vi "Measurement UI.vi"() -> ()   [LabVIEW 2023, in "FPT_Compression UI.lvlib"]
uses:
  FPT_Compression UI.lvlib
panel:
  in  "Measurement Graph":T1(tab)
  out "General Graph 1":T2(graph)
  out "General Graph 2":T2(graph)
  out "General Graph 3":T2(graph)
  out "General Graph 4":T2(graph)
  out "General Graph 5":T2(graph)
  out "PAE@Pin(s)":string[](array[string])
  out "Gain@Pin(s)":string[](array[string])
  out "Pout@Pin(s)":string[](array[string])
  out "Pout@Pin vs Freq":dbl[][](array[numeric])
  out "PAE vs Pin per Freq":dbl[][](array[numeric])
  in  "RFSG attenuation s2p path name":string caption="RFSG ATTENUATION S2P PATH NAME"
  in  "RFmx attenuation s2p path name":string caption="RFmx ATTENUATION S2P PATH NAME"
  in  "RFSG attenuation path name":string caption="RFSG ATTENUATION PATH NAME"
  in  "RFmx attenuation path name":string caption="RFmx ATTENUATION PATH NAME"
  out "Gain vs Pin per Freq":dbl[][](array[numeric])
  out "Group B Graph":refnum<vi>[](array[refnum])
  out "Group A Graph":refnum<vi>[](array[refnum])
  in  "Power sequencing file path":string
  in  "RFSG name":string="5842_0"
  in  "RFSG attenuation mode":T3(ring)=enum."s2p File"
  in  "RFSG s2p file path":string
  in  "RFmx name":string="5842_0"
  in  "RFmx attenuation mode":T3(ring)=enum."Constant Attenuation"
  in  "RFmx s2p file path":string
  out "All Graph Refs":refnum<vi>[](array[refnum])
  out "Pout vs Pin per Freq":dbl[][](array[numeric])
  out "OPxdB vs Freq":dbl[][](array[numeric])
  out "Linear Gain vs Freq":dbl[][](array[numeric])
  out "Frequencies":string[](array[string])
  out "OPxdB(s)":string[](array[string])
  out "Linear Gain(s)":string[](array[string])
  out "Full Data per Frequency":string[][](array[string])
  out "Pin(s)":string[](array[string])
  in  "Compression_Stimulus Mode":T4(ring)
  in  "SMU name":string caption="SMU Name"
  out "Table 2 Header":string[](array[string])
  out "Table 1 Header":string[](array[string])
  out "Gain@Pin vs Freq":dbl[][](array[numeric])
  out "PAE@Pin vs Freq":dbl[][](array[numeric])
  out "MeasTable 1":string[][](table)
  out "MeasTable 2":string[][](table)
  in  "Mode of operation":T5(ring) caption="Configuration"
  in  "Tab Control":T6(tab)
  in  "Power sequencing file path_update":path caption="Power Sequencing File Path"
  in  "SMU channel":string caption="SMU Channel"
  in  "SMU name_update":refnum<k15> caption="SMU Name"
  in  "RFmx port":string(combo)="port2" caption="RFmx Port"
  in  "RFSG port":string(combo)="port1" caption="RFSG Port"
  in  "RFSG name_update":refnum<k15> caption="RFSG Name"
  in  "RFSG attenuation mode_tab":T3(tab)=enum."s2p File" caption="RFSG Attenuation Mode"
  in  "RFSG external attenuation (dB)":dbl caption="External Attenuation" format="%#.3fdB"
  in  "RFSG s-parameters orientation":enum32{"Port1 Towards DUT", "Port2 Towards DUT"}(ring) caption="Orientation"
  in  "RFSG s2p file path_update":path caption="S2P File Path"
  in  "RFmx attenuation mode_tab":T3(tab)=enum."s2p File" caption="RFmx Attenuation Mode"
  in  "RFmx external attenuation (dB)":dbl caption="External Attenuation" format="%#.3fdB"
  in  "RFmx s2p file path_update":path caption="S2P File Path"
  in  "RFmx s-parameters orientation":enum32{"Port1 Towards DUT", "Port2 Towards DUT"}(ring) caption="Orientation"
  in  "RFmx name_update":refnum<k15> caption="RFmx Name"
  in  "DC & RF Mode":T4(tab)
  in  "CP_CW_DC Source Delay (s)":dbl caption="DC Source Delay" format="%#ps"
  in  "CP_PRF_RFmx Trigger Delay (s)":dbl caption="RFmx Trigger Delay" format="%#ps"
  in  "CP_PRF_PRI (s)":dbl=0.001 caption="PRI" format="%#ps"
  in  "CP_PRF_RF Pulse Width (s)":dbl=0.0001 caption="RF Pulse Width" format="%#ps"
  in  "CP_PRF_DC Source Delay (s)":dbl caption="DC Source Delay" format="%#ps"
  in  "PP_PRF_ON Current Limit (A)":dbl=0.2 caption="Pulse ON Current Limit" format="%#pA"
  in  "PP_PRF_PRI (s)":dbl=0.001 caption="PRI" format="%#ps"
  in  "PP_PRF_RF Pulse Width (s)":dbl=0.0001 caption="RF Pulse Width" format="%#ps"
  in  "PP_PRF_DC Source Delay (s)":dbl caption="DC Source Delay" format="%#ps"
  in  "PP_PRF_RFmx Trigger Delay (s)":dbl caption="RFmx Trigger Delay" format="%#ps"
  in  "PP_PRF_DC Pulse Width (s)":dbl=0.0008 caption="DC Pulse Width" format="%#ps"
  in  "PP_PRF_Bias Voltage Level (V)":dbl caption="Pulse OFF Voltage Level" format="%#pV"
  in  "PP_PRF_Bias Current Limit (A)":dbl=0.2 caption="Pulse OFF Current Limit" format="%#pA"
  in  "Compression_DC Measurement Interval (s)":dbl=5e-05 caption="DC Measurement Interval" format="%#ps"
  in  "Compression_RF Measurement Interval (s)":dbl=5e-05 caption="RF Measurement Interval" format="%#ps"
  in  "Compression_Target Pin (dBm)":dbl=1.0 caption="Target Pin" format="%#pdBm"
  in  "Compression_Expected DUT Gain (dB)":dbl=17.5 caption="Expected DUT Gain" format="%#pdB"
  in  "Compression_Max Linear Range (dBm)":dbl=-10.0 caption="Max Linear Range" format="%#pdBm"
  in  "Compression_Compression Point (dB)":dbl=1.0 caption="PxdB" format="%#pdB"
  in  "Compression_RFSG Frequency Start (Hz)":dbl=6000000000.0 caption="Frequency Start" step=1000000.0 format="%#pHz"
  in  "Compression_RFSG Power Start (dBm)":dbl=-20.0 caption="Power Start" format="%#pdBm"
  in  "Compression_RFSG Power Step Size (dB)":dbl=1.0 caption="Power Step Size" format="%#pdB"
  in  "Compression_RFSG Power Stop(dBm)":dbl=4.0 caption="Power End" format="%#pdBm"
  in  "Compression_RBW (Hz)":dbl=5000000.0 caption="RBW" format="%#pHz"
  in  "Compression_RFSG Frequency Stop (Hz)":dbl=18000000000.0 caption="Frequency Stop" step=1000000.0 format="%#pHz"
  in  "Compression_RFSG Number of Frequency Step":i32=10 caption="Number of Steps"
  out "Status":string
  # "Frequency Sweep"
  # "Power Sweep"
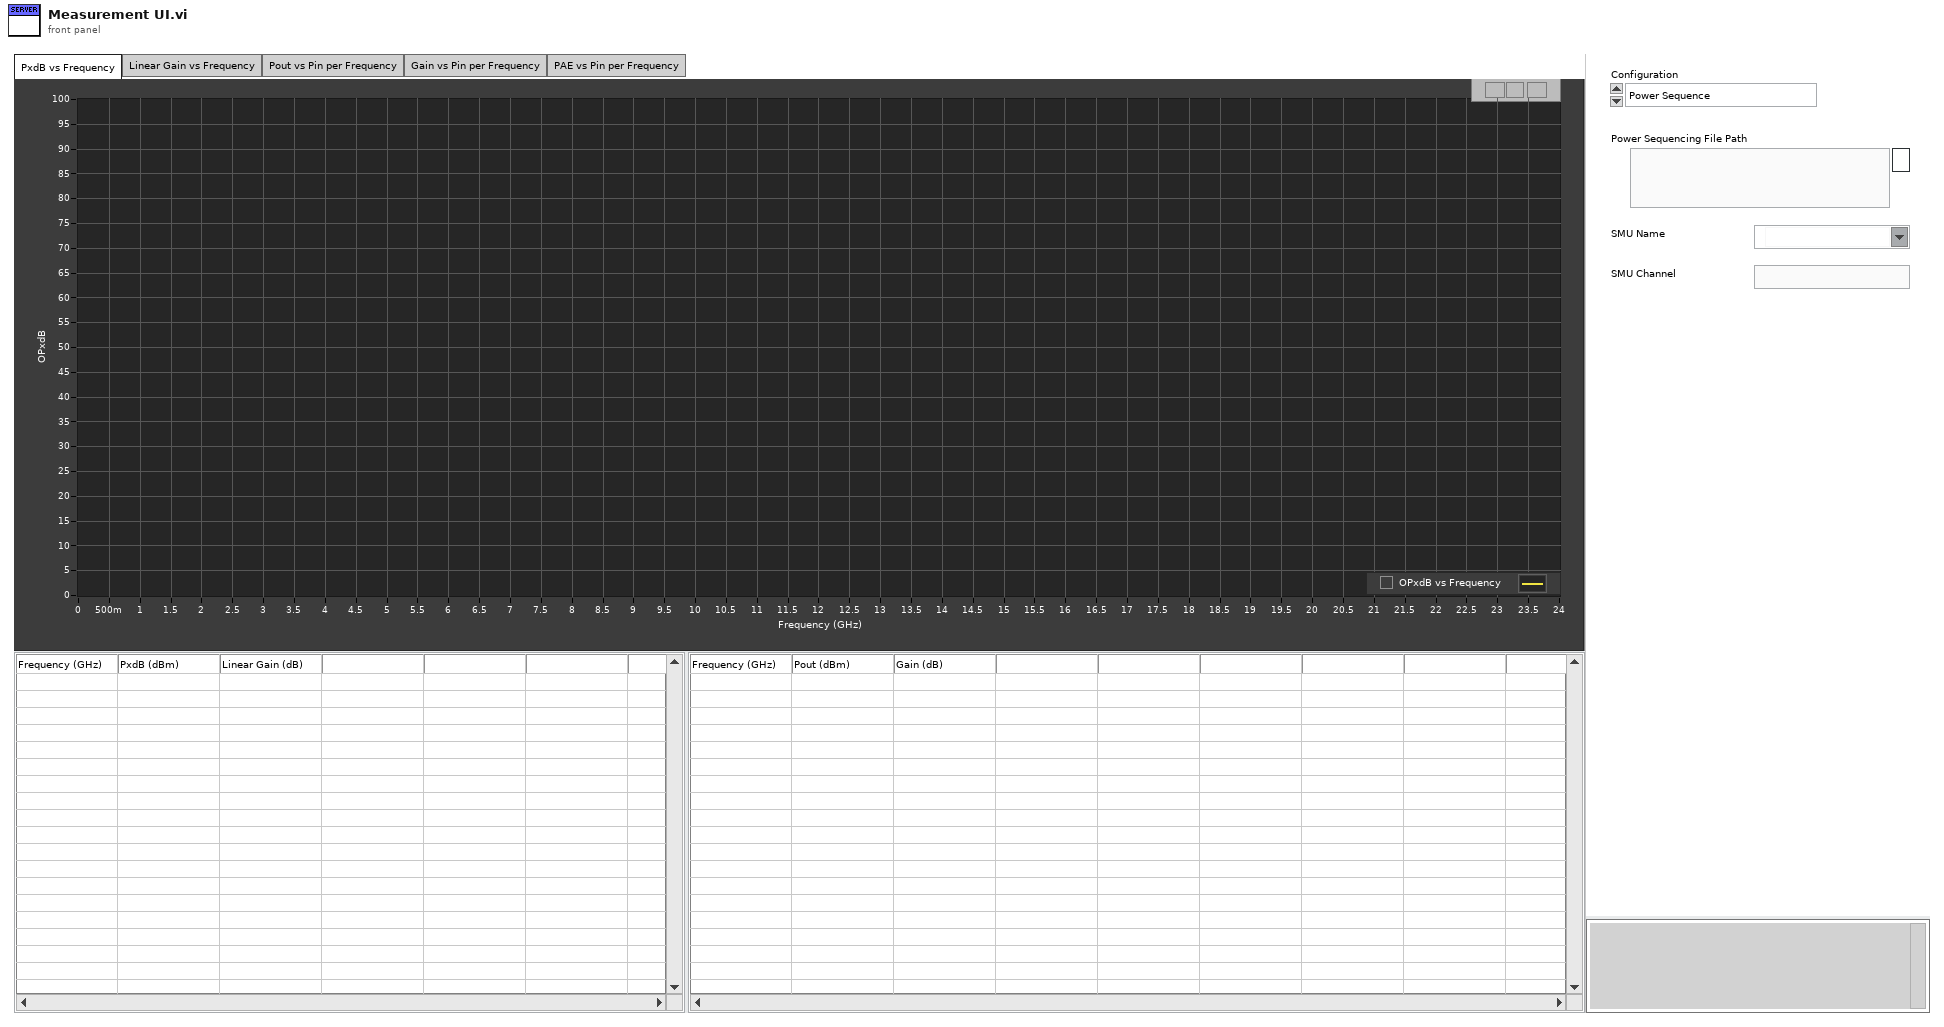
[diagram p1: front panel]
types:
  T1 = enum32{"PxdB vs Frequency", "Linear Gain vs Frequency", "Pout vs Pin per Frequency", "Gain vs Pin per Frequency", "PAE vs Pin per Frequency", "Hidden Controls"}
  T2 = cluster{"Load currents":dbl[], "Efficiency":dbl[]}[]
  T3 = enum32{"<None>", "Constant Attenuation", "s2p File"}
  T4 = enum32{"Constant Power and RF", "Constant Power and Pulsed RF", "Pulsed Power and RF"}
  T5 = enum32{"Power Sequence", "HW + Correction", "Mode", "Measurement 1"}
  T6 = enum32{"Power Sequence", "Correction", "Mode", "Measurement 1"}
  T7 = enum16{"<None>", "Constant Attenuation", "s2p File"}
  T8 = cluster{"Shift":bool, "Ctrl":bool, "Alt":bool, "Cmd":bool, "Opt":bool}
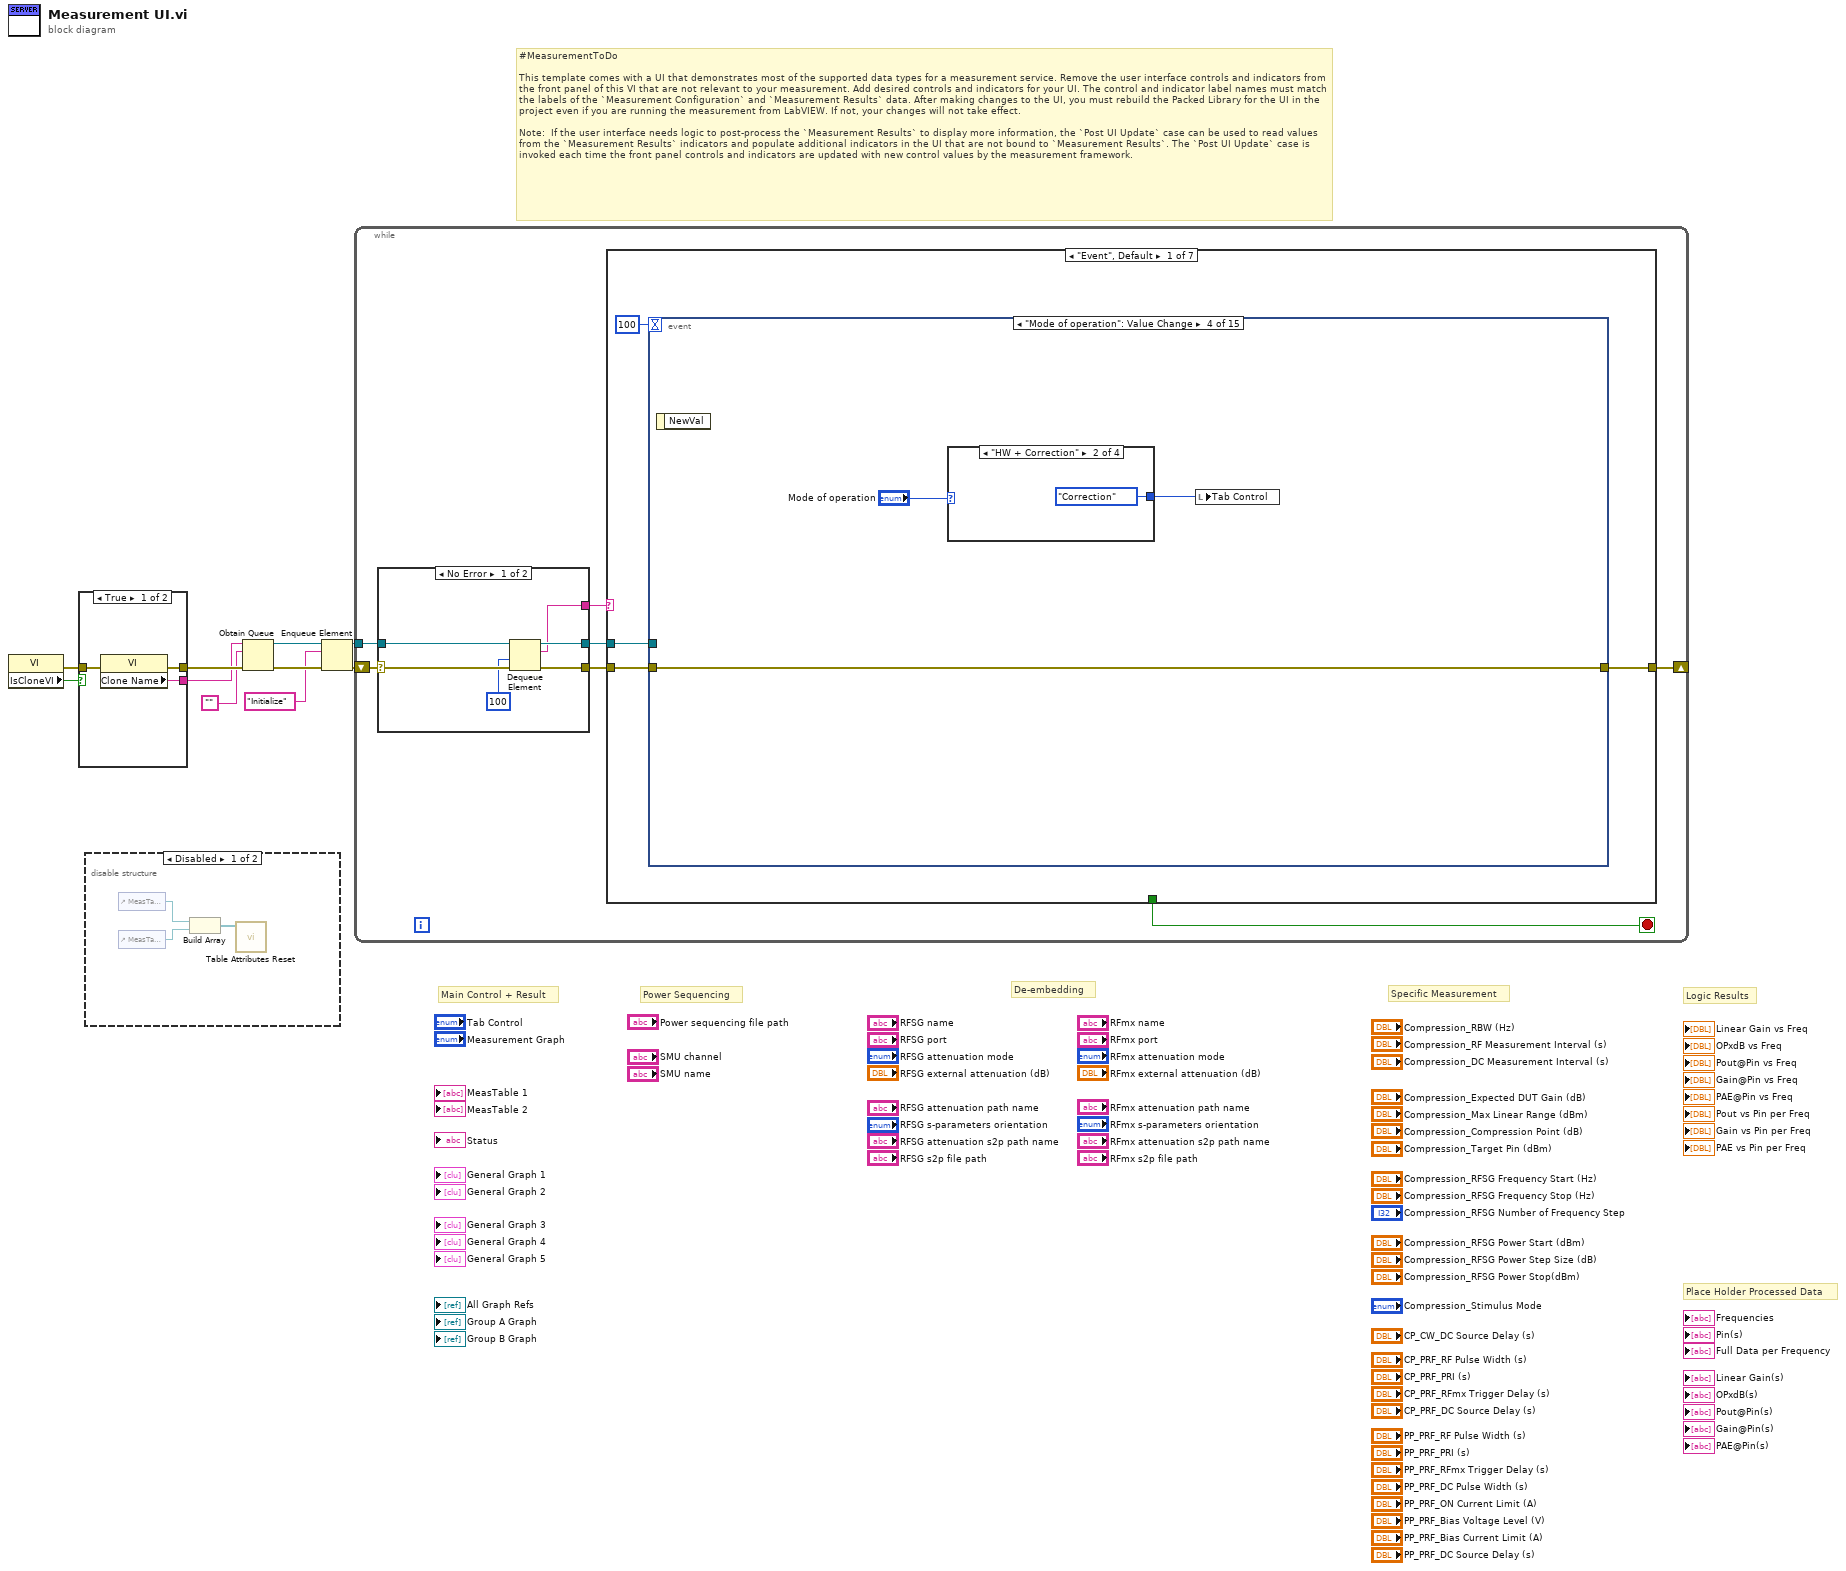
[diagram p0: block diagram]
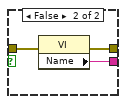
[diagram p3: hidden frame]
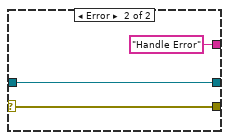
[diagram p4: hidden frame]
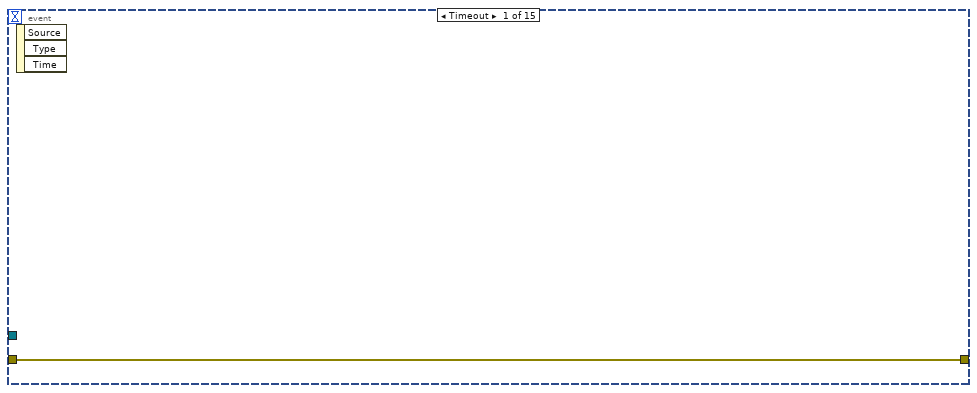
[diagram p5: hidden frame]
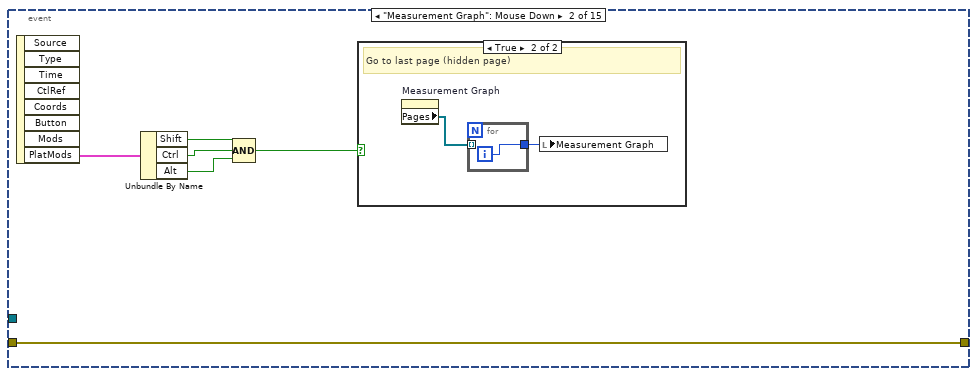
[diagram p6: hidden frame]
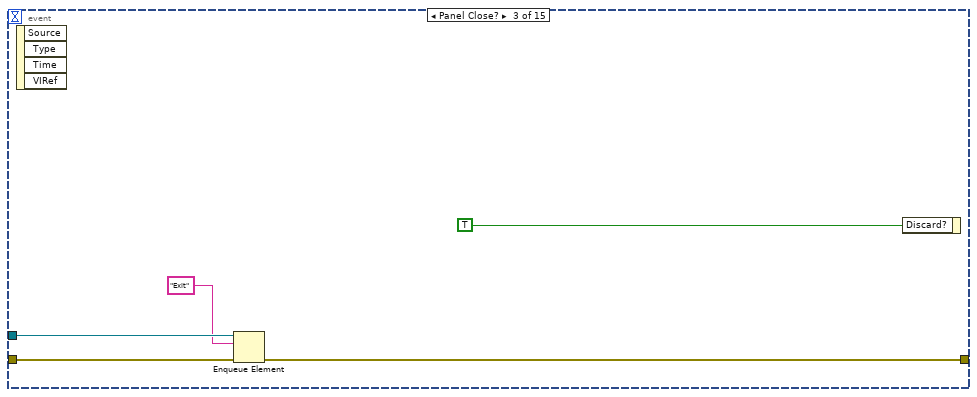
[diagram p8: hidden frame]
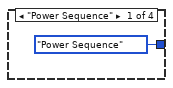
[diagram p9: hidden frame]
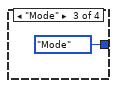
[diagram p10: hidden frame]
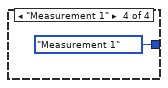
[diagram p11: hidden frame]
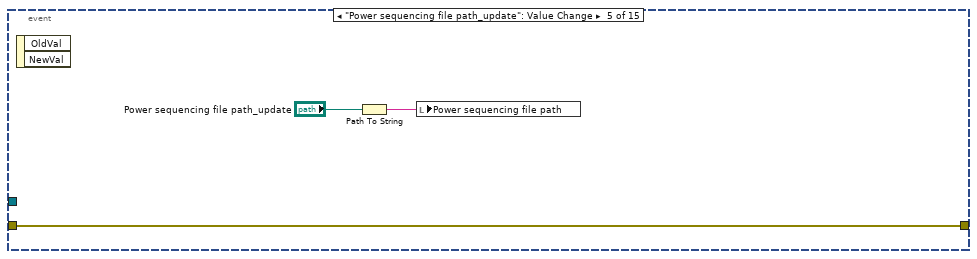
[diagram p12: hidden frame]
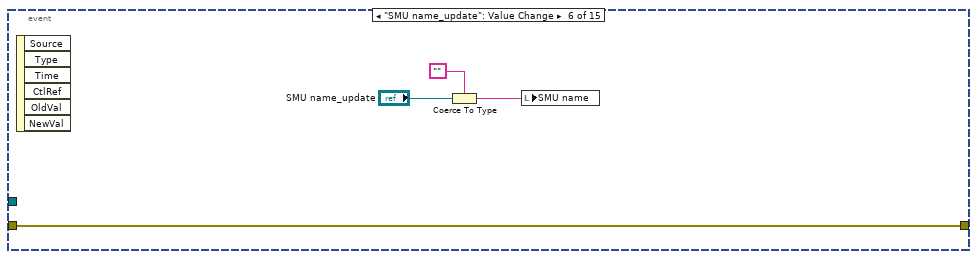
[diagram p13: hidden frame]
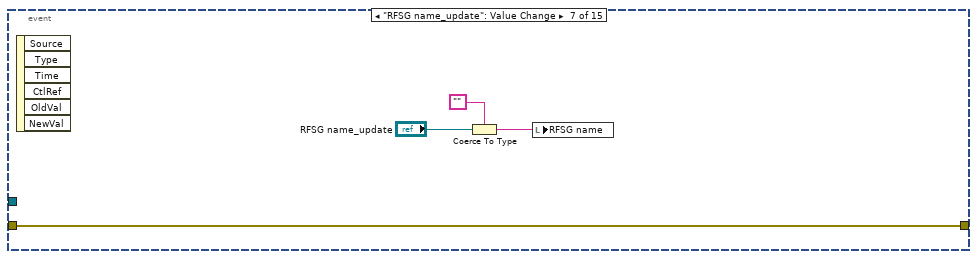
[diagram p14: hidden frame]
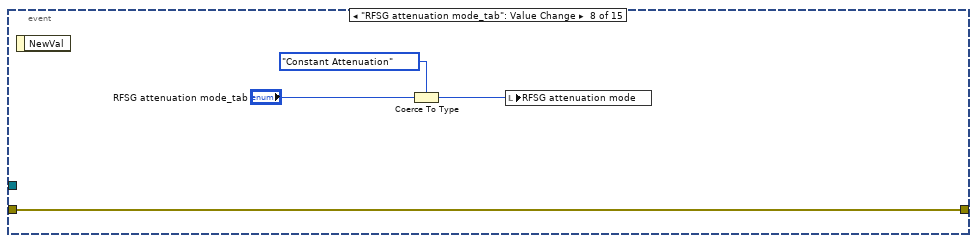
[diagram p15: hidden frame]
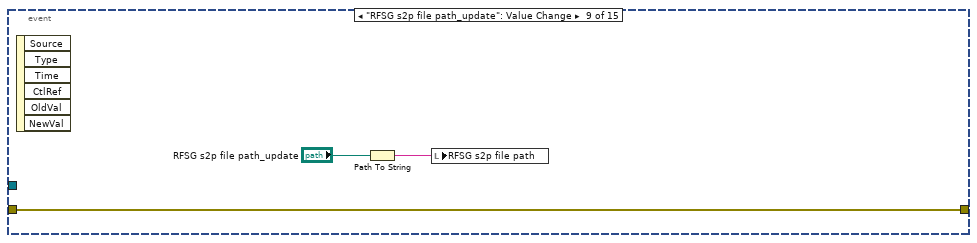
[diagram p16: hidden frame]
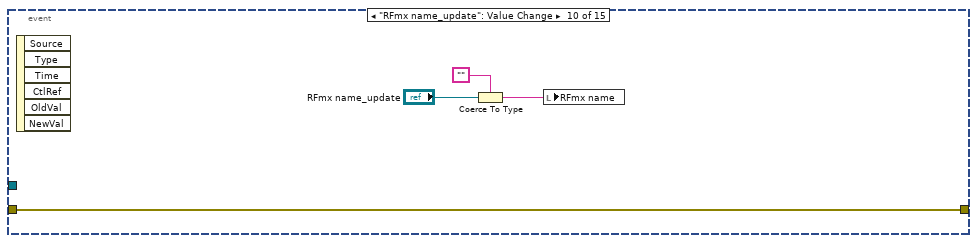
[diagram p17: hidden frame]
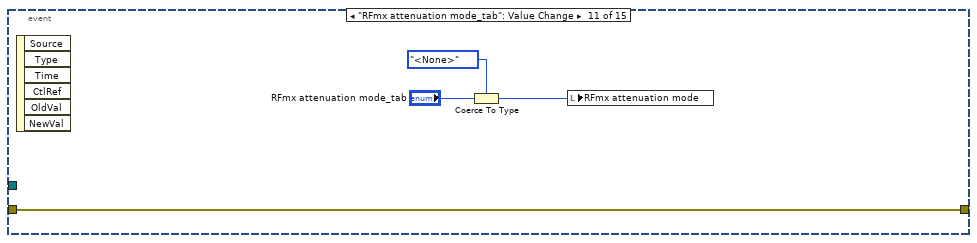
[diagram p18: hidden frame]
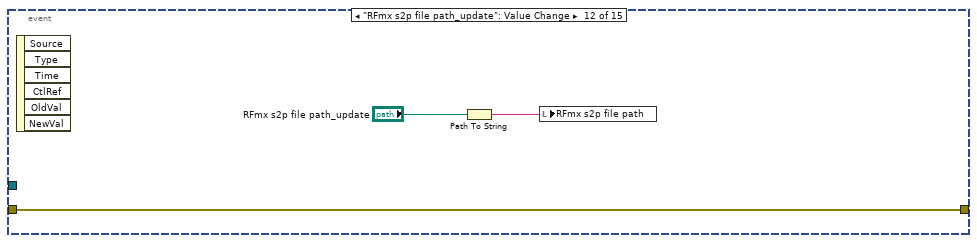
[diagram p19: hidden frame]
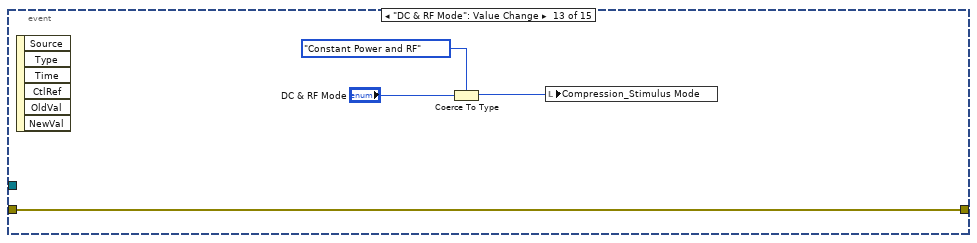
[diagram p20: hidden frame]
diagram:
  # "Logic Results"
  # "Place Holder Processed Data"
  # "Specific Measurement"
  # "De-embedding"
  # "Power Sequencing"
  # "Main Control + Result"
  # "#MeasurementToDo  \n\nThis template comes with a UI that demonstrates most of the supported data types for a measurement service. Remove the user interface controls and indicators from the front panel of this VI that are not relevant to your measurement. Add desired controls and indicators for your UI. The control and indicator label names must match the labels of the `Measurement Configuration` and `Measurement Results` data. After making changes to the UI, you must rebuild the Packed Library for the UI in the project even if you are running the measurement from LabVIEW. If not, your changes will not take effect.\n\nNote:  If the user interface needs logic to post-process the `Measurement Results` to display more information, the `Post UI Update` case can be used to read values from the `Measurement Results` indicators and populate additional indicators in the UI that are not bound to `Measurement Results`. The `Post UI Update` case is invoked each time the front panel controls and indicators are updated with new control values by the measurement framework."
  n1 = property class="VI"() -> (error out=w1:errorcluster, "IsCloneVI"=w2:bool)  [unwired: 2 in, 1 out]
  n2 = case shown="True" w2 {
    tunnel: [w13 w16] -> w10
    tunnel: [w12 w15] -> w9
    tunnel: w1 -> [w11 w14]
    frame True {
      n3 = property class="VI"(error in=w11) -> (error out=w13:errorcluster, "Clone Name"=w12:string)  [unwired: 1 in, 1 out]
    }
    frame False {
      n4 = property class="VI"(error in=w14) -> (error out=w16:errorcluster, "Name"=w15:string)  [unwired: 1 in, 1 out]
    }
  }
  n5 = disable-structure shown="Disabled" {
    frame Disabled {
      n6 = control-ref of="MeasTable 2"() -> (w19:refnum<vi>)
      n7 = control-ref of="MeasTable 1"() -> (w18:refnum<vi>)
      n8 = Build Array(w19, w18) -> (w17:refnum<vi>[])
      n9 = call "Table Attributes Reset.vi"("Table Refs"=w17) -> ()  [unwired: 11 in]
    }
    frame Enabled {
    }
  }
  n10 = Obtain Queue(name (unnamed)=w9, element data type="", error in (no error)=w10) -> (queue out=w6:refnum<queue>, error out=w8:errorcluster)  [unwired: 2 in, 1 out]
  n11 = Enqueue Element(queue=w6, element="Initialize", error in (no error)=w8) -> (queue out=w5:refnum<queue>, error out=w7:errorcluster)  [unwired: 1 in, 1 out]
  n12 = while {
    shift-right: [w21] -> _
    shift-left: w7 -> [w26]
    tunnel: w5 -> [w24]
    stop <- w20 stop-if-true
    n13 = case shown="No Error" w26 {
      selector: w26 -> [w32 w35]
      tunnel: [w31 w35] -> w25
      tunnel: w24 -> [w30 w34]
      tunnel: [w29 w34] -> w23
      tunnel: [w28 "Handle Error"] -> w22
      frame No Error {
        n14 = Dequeue Element(queue=w30, timeout in ms (-1)=100, error in (no error)=w32) -> (queue out=w29:refnum<queue>, element=w28:string, error out=w31:errorcluster)  [unwired: 1 out]
      }
      frame Error {
      }
    }
    n15 = case shown="\"Event\", Default" w22 {
      tunnel: w25 -> [w38 w150 w217 w259 w267 w274 w275]
      tunnel: w23 -> [w36 _ w216 w257 _ w272 _]
      tunnel: [w39 w150 w217 w258 w262 w269 w275] -> w21
      tunnel: [_ _ _ _ _ TRUE _] -> w20
      frame "Event", Default {
        n16 = event shown="[3] \"Mode of operation\": Value Change" {
          selector: _ -> [_ _ _ _ _ _ _ _ _ _ _ _ _ _ _]
          dyn-events: _ -> [_ _ _ _ _ _ _ _ _ _ _ _ _ _ _]
          timeout: 100 -> [_ _ _ _ _ _ _ _ _ _ _ _ _ _ _]
          tunnel: [w40 w41 w52 w56 w62 w68 w69 w73 w77 w80 w84 w88 w94 w107 w128] -> w39
          tunnel: w38 -> [w40 w41 w53 w56 w62 w68 w69 w73 w77 w80 w84 w88 w94 w109 w129]
          tunnel: w36 -> [_ _ w51 _ _ _ _ _ _ _ _ _ _ _ _]
          event Timeout {
            n17 = event-data() -> ()  [unwired: 1 in, 3 out]
          }
          event "Measurement Graph": Mouse Down {
            n18 = event-data() -> ("PlatMods"=w46:T8)  [unwired: 1 in, 7 out]
            n19 = Unbundle By Name(w46) -> ("Shift"=w45:bool, "Ctrl"=w44:bool, "Alt"=w43:bool)
            n20 = Compound Arithmetic op=AND(w45, w44, w43) -> (w42:bool)
            n21 = case shown="True" w42 {
              frame False {
              }
              frame True {
                # "Go to last page (hidden page)"
                n22 = property on="Measurement Graph" class="TabCtl (strict)"() -> ("Pages"=w48:refnum<vi>[])  [unwired: 2 in, 2 out]
                n23 = for {
                  tunnel: w48 -> [_] mode=indexing
                  tunnel: [w49] -> w47
                  i -> [w49]
                }
                n24 = local write "Measurement Graph"(w47) -> ()
              }
            }
          }
          event Panel Close? {
            n25 = event-data() -> ()  [unwired: 1 in, 4 out]
            n26 = Enqueue Element(queue=w51, element="Exit", error in (no error)=w53) -> (error out=w52:errorcluster)  [unwired: 1 in, 2 out]
            n27 = event-data("Discard?"=TRUE) -> ()  [unwired: 1 in, 1 out]
          }
          event "Mode of operation": Value Change {
            n28 = event-data() -> ()  [unwired: 1 in, 1 out]
            n29 = case shown="\"HW + Correction\"" "Mode of operation" {
              tunnel: [T6."Power Sequence" ("Tab Control") T6."Correction" ("Tab Control") T6."Mode" ("Tab Control") T6."Measurement 1" ("Tab Control")] -> w55
              frame "Power Sequence" {
              }
              frame "HW + Correction" {
              }
              frame "Mode" {
              }
              frame "Measurement 1" {
              }
            }
            n30 = local write "Tab Control"(w55) -> ()
          }
          event "Power sequencing file path_update": Value Change {
            n31 = event-data() -> ()  [unwired: 1 in, 2 out]
            n32 = Path To String(path="Power sequencing file path_update") -> (string=w63:string)
            n33 = local write "Power sequencing file path"(w63) -> ()
          }
          event "SMU name_update": Value Change {
            n34 = event-data() -> ()  [unwired: 1 in, 6 out]
            n35 = Coerce To Type(0:"SMU name_update", 1:"") -> (2:w65:string)
            n36 = local write "SMU name"(w65) -> ()
          }
          event "RFSG name_update": Value Change {
            n37 = event-data() -> ()  [unwired: 1 in, 6 out]
            n38 = Coerce To Type(0:"RFSG name_update", 1:"") -> (2:w70:string)
            n39 = local write "RFSG name"(w70) -> ()
          }
          event "RFSG attenuation mode_tab": Value Change {
            n40 = event-data() -> ()  [unwired: 1 in, 1 out]
            n41 = Coerce To Type(0:"RFSG attenuation mode_tab", 1:T3."Constant Attenuation" ("RFSG attenuation mode")) -> (2:w75:T3)
            n42 = local write "RFSG attenuation mode"(w75) -> ()
          }
          event "RFSG s2p file path_update": Value Change {
            n43 = event-data() -> ()  [unwired: 1 in, 6 out]
            n44 = Path To String(path="RFSG s2p file path_update") -> (string=w78:string)
            n45 = local write "RFSG s2p file path"(w78) -> ()
          }
          event "RFmx name_update": Value Change {
            n46 = event-data() -> ()  [unwired: 1 in, 6 out]
            n47 = Coerce To Type(0:"RFmx name_update", 1:"") -> (2:w82:string)
            n48 = local write "RFmx name"(w82) -> ()
          }
          event "RFmx attenuation mode_tab": Value Change {
            n49 = event-data() -> ()  [unwired: 1 in, 6 out]
            n50 = Coerce To Type(0:"RFmx attenuation mode_tab", 1:T7."<None>" ("RFmx attenuation mode")) -> (2:w85:T7)
            n51 = local write "RFmx attenuation mode"(w85) -> ()
          }
          event "RFmx s2p file path_update": Value Change {
            n52 = event-data() -> ()  [unwired: 1 in, 6 out]
            n53 = Path To String(path="RFmx s2p file path_update") -> (string=w89:string)
            n54 = local write "RFmx s2p file path"(w89) -> ()
          }
          event "DC & RF Mode": Value Change {
            n55 = event-data() -> ()  [unwired: 1 in, 6 out]
            n56 = Coerce To Type(0:"DC & RF Mode", 1:T4."Constant Power and RF" ("Compression_Stimulus Mode")) -> (2:w92:T4)
            n57 = local write "Compression_Stimulus Mode"(w92) -> ()
          }
          event "General Graph 1", "General Graph 2": Cursor Move {
            n58 = event-data() -> ("CtlRef"=w100:refnum<vi>, "PointIdx"=w106:i32, "CursLoc"=w104:cluster{"X":dbl, "Y":dbl})  [unwired: 1 in, 6 out]
            n59 = Unbundle By Name(w104) -> ("X"=w103:dbl)
            n60 = property on="Group A Graph" class="Arr (strict)"() -> ("Value"=w101:refnum<vi>[])  [unwired: 2 in, 2 out]
            n61 = Search 1D Array(1D array=w101, element=w100) -> (index of element=w102:i32)  [unwired: 1 in]
            n62 = Delete From Array(array=w101, index=w102) -> (array with subset deleted=w99:refnum<vi>[])  [unwired: 1 in, 1 out]
            n63 = call "Graph Cursor Update.vi"("Action"=enum16{"Reset", "Update"}."Update", "error in"=w109, "New X position"=w103, "Cursor Type"=enum16{"Movable", "Fixed", "All"}."Movable", "Graph Refs in"=w99) -> ("error out"=w108:errorcluster)  [unwired: 5 in, 1 out]
            n64 = control-ref of="MeasTable 1"() -> (w96:refnum<vi>)
            n65 = call "Table Highlight.vi"("Action"=enum16{"Reset", "Highlight 1 Row"}."Highlight 1 Row", "error in"=w108, "Color Box"=u32 16776960, "Row"=w106, "Table Ref in"=w96) -> ("error out"=w107:errorcluster)  [unwired: 5 in, 1 out]
          }
          event "General Graph 3", "General Graph 4", "General Graph 5": Cursor Move {
            # "------------------------Table2------------------------\n<Freq><Pin><Pout><Gain><PAE>"
            n66 = event-data() -> ("CtlRef"=w122:refnum<vi>, "PointIdx"=w112:i32, "CursLoc"=w126:cluster{"X":dbl, "Y":dbl})  [unwired: 1 in, 6 out]
            n67 = Unbundle By Name(w126) -> ("X"=w125:dbl)
            n68 = property on="Group B Graph" class="Arr (strict)"() -> ("Value"=w123:refnum<vi>[])  [unwired: 2 in, 2 out]
            n69 = Search 1D Array(1D array=w123, element=w122) -> (index of element=w124:i32)  [unwired: 1 in]
            n70 = Delete From Array(array=w123, index=w124) -> (array with subset deleted=w121:refnum<vi>[])  [unwired: 1 in, 1 out]
            n71 = call "Graph Cursor Update.vi"("Action"=enum16{"Reset", "Update"}."Update", "error in"=w129, "New X position"=w125, "Cursor Type"=enum16{"Movable", "Fixed", "All"}."Movable", "Graph Refs in"=w121) -> ("error out"=w128:errorcluster)  [unwired: 5 in, 1 out]
            n72 = local read "Frequencies"() -> (w113:string[])
            n73 = local read "Pin(s)"() -> (w116:string[])
            n74 = Index Array(array=w116, index=w112) -> (element=w115:string)
            n75 = local read "Full Data per Frequency"() -> (w117:string[][])
            n76 = local read "Table 2 Header"() -> (w110:string[])
            n77 = for {
              tunnel: [w130] -> w114 mode=indexing
              tunnel: w115 -> [w130]
              tunnel: w113 -> [_] mode=indexing
            }
            n78 = control-ref of="MeasTable 2"() -> (w119:refnum<vi>)
            n79 = call "Get Data per Frequency at Pin Point Index.vi"("Pin Point Index"=w112, "Full Data per Freq"=w117) -> ("Focused Data"=w111:string[][])  [unwired: 9 in]
            n80 = Build Array (concatenate)(w113, w114, w111) -> (w118:string[][])
            n81 = call "Table Set Header Name and Data (String).vi"("Data"=w118, "Header"=w110, "Table Ref"=w119) -> ()  [unwired: 9 in]
          }
        }
      }
      frame "Initialize" {
        w142 = 0
        # "-------Go to Default Page/Tab-------"
        # "-------------------------Assign Graph References in Group-------------------------"
        n82 = local write "Tab Control"(w142) -> ()
        n83 = local write "Mode of operation"(w142) -> ()
        n84 = local write "Measurement Graph"(w142) -> ()
        n85 = control-ref of="General Graph 1"() -> (w145:refnum<vi>)
        n86 = control-ref of="General Graph 2"() -> (w144:refnum<vi>)
        n87 = control-ref of="General Graph 3"() -> (w143:refnum<vi>)
        n88 = control-ref of="General Graph 4"() -> (w134:refnum<vi>)
        n89 = control-ref of="General Graph 5"() -> (w133:refnum<vi>)
        n90 = Build Array(w145, w144, w143, w134, w133) -> (w141:refnum<vi>[])
        n91 = Build Array(w145, w144) -> (w140:refnum<vi>[])
        n92 = Build Array(w143, w134, w133) -> (w135:refnum<vi>[])
        n93 = local write "All Graph Refs"(w141) -> ()
        n94 = local write "Group A Graph"(w140) -> ()
        n95 = call "Graph Set Cursor Mode.vi"("Cursor Mode"=enum32{"Free-Drag", "Single-Plot", "Multi-Plot"}."Single-Plot", "Graph Refs in"=w140) -> ("Graph Refs out"=w146:refnum<vi>[])  [unwired: 8 in, 1 out]
        n96 = call "Graph Set Cursor Mode.vi"("Cursor Mode"=enum32{"Free-Drag", "Single-Plot", "Multi-Plot"}."Multi-Plot", "Graph Refs in"=w135) -> ("Graph Refs out"=w139:refnum<vi>[])  [unwired: 8 in, 1 out]
        n97 = local write "Group B Graph"(w135) -> ()
        n98 = call "Graph Cursor Update.vi"("Action"=enum16{"Reset", "Update"}."Reset", "Cursor Type"=enum16{"Movable", "Fixed", "All"}."All", "Graph Refs in"=w146) -> ()  [unwired: 7 in, 2 out]
        n99 = call "Graph Cursor Update.vi"("Action"=enum16{"Reset", "Update"}."Reset", "Cursor Type"=enum16{"Movable", "Fixed", "All"}."All", "Graph Refs in"=w139) -> ()  [unwired: 7 in, 2 out]
        "Table 2 Header" <- string[] ["Frequency (GHz)", "Pin (dBm)", "Pout (dBm)", "Gain (dB)", "PAE (%)"] ("Header")
        "Table 1 Header" <- string[] ["Frequency (GHz)", "PxdB (dBm)", "Linear Gain (dB)", "Pout@Target Pin", "Gain@Target Pin", "PAE@Target Pin"] ("Header")
      }
      frame "Post UI Update" {
        # "--------------------Get Pout@Pin--------------------"
        # "------------------Get PAE@Pin--------------------"
        # "--------------------Get Gain@Pin--------------------"
        # "------------Get Pout(s) and Gain(s) per Frequency------------"
        # "-------------------------Get Frequencies-------------------------"
        # "------------------Get Linear Gain------------------"
        # "--------------------Get OPxdB--------------------"
        # "--------------------Get Pin(s)--------------------"
        # "This case will be triggered, after framework updates the User interface with result values.\nUsed to update data type def"
        n100 = local read "Power sequencing file path"() -> (w213:string)
        n101 = local read "Compression_Stimulus Mode"() -> (w172:T4)
        n102 = local read "RFSG attenuation mode"() -> (w212:T3)
        n103 = local read "RFmx attenuation mode"() -> (w198:T3)
        n104 = local read "SMU name"() -> (w170:string)
        n105 = local read "RFSG s2p file path"() -> (w205:string)
        n106 = local read "RFmx s2p file path"() -> (w204:string)
        n107 = local read "RFSG name"() -> (w209:string)
        n108 = local read "RFmx name"() -> (w200:string)
        n109 = Enqueue Element(queue=w216, element="Post UI Update 2") -> ()  [unwired: 2 in, 3 out]
        n110 = Coerce To Type(0:w170, 1:refnum<k15> refnum ("RFSG name_update")) -> (2:w168:refnum<k15>)
        n111 = Coerce To Type(0:w172, 1:T4."Constant Power and RF" ("DC & RF Mode")) -> (2:w171:T4)
        n112 = local write "SMU name_update"(w168) -> ()
        n113 = Coerce To Type(0:w212, 1:T3."<None>" ("RFSG attenuation mode_tab")) -> (2:w211:T3)
        n114 = Coerce To Type(0:w200, 1:refnum<k15> refnum ("RFSG name_update")) -> (2:w202:refnum<k15>)
        n115 = String To Path(string=w204) -> (path=w203:path)
        n116 = Coerce To Type(0:w209, 1:refnum<k15> refnum ("RFSG name_update")) -> (2:w207:refnum<k15>)
        n117 = Coerce To Type(0:w198, 1:T3."<None>" ("RFmx attenuation mode_tab")) -> (2:w199:T3)
        n118 = String To Path(string=w213) -> (path=w214:path)
        n119 = String To Path(string=w205) -> (path=w206:path)
        n120 = local write "DC & RF Mode"(w171) -> ()
        n121 = local write "RFmx name_update"(w202) -> ()
        n122 = local write "RFmx attenuation mode_tab"(w199) -> ()
        n123 = local write "RFmx s2p file path_update"(w203) -> ()
        n124 = local write "Power sequencing file path_update"(w214) -> ()
        n125 = local write "RFSG name_update"(w207) -> ()
        n126 = local write "RFSG attenuation mode_tab"(w211) -> ()
        n127 = local write "RFSG s2p file path_update"(w206) -> ()
        n128 = local read "Pout vs Pin per Freq"() -> (w193:dbl[][])
        n129 = local read "Linear Gain vs Freq"() -> (w187:dbl[][])
        n130 = local read "OPxdB vs Freq"() -> (w189:dbl[][])
        n131 = Index Array(array=w193) -> (element=w192:dbl[])  [unwired: 2 in]
        n132 = Index Array(array=w189, index (row)=1) -> (element=w186:dbl[])  [unwired: 1 in]
        n133 = Index Array(array=w187, index (row)=1) -> (element=w184:dbl[])  [unwired: 1 in]
        n134 = local read "Gain vs Pin per Freq"() -> (w178:dbl[][])
        n135 = local read "PAE vs Pin per Freq"() -> (w164:dbl[][])
        n136 = local read "Pout vs Pin per Freq"() -> (w177:dbl[][])
        n137 = Number To Fractional String(number=w192) -> (F-format string=w191:string[])  [unwired: 3 in]
        n138 = Number To Fractional String(number=w186) -> (F-format string=w185:string[])  [unwired: 3 in]
        n139 = Number To Fractional String(number=w184) -> (F-format string=w183:string[])  [unwired: 3 in]
        n140 = local write "Pin(s)"(w191) -> ()
        n141 = local write "OPxdB(s)"(w185) -> ()
        n142 = local write "Linear Gain(s)"(w183) -> ()
        n143 = Delete From Array(array=w177, length=1, index (row)=0) -> (array with subset deleted=w179:dbl[][])  [unwired: 1 in, 1 out]
        n144 = Delete From Array(array=w178, length=1, index (row)=0) -> (array with subset deleted=w180:dbl[][])  [unwired: 1 in, 1 out]
        n145 = Delete From Array(array=w164, length=1, index (row)=0) -> (array with subset deleted=w163:dbl[][])  [unwired: 1 in, 1 out]
        n146 = local read "Linear Gain vs Freq"() -> (w196:dbl[][])
        n147 = Build Array (concatenate)(w179, w180, w163) -> (w181:dbl[][])
        n148 = local read "Pout@Pin vs Freq"() -> (w153:dbl[][])
        n149 = local read "Gain@Pin vs Freq"() -> (w156:dbl[][])
        n150 = local read "PAE@Pin vs Freq"() -> (w158:dbl[][])
        n151 = Number To Fractional String(number=w181) -> (F-format string=w182:string[][])  [unwired: 3 in]
        n152 = local write "Full Data per Frequency"(w182) -> ()
        n153 = Index Array(array=w196) -> (element=w195:dbl[])  [unwired: 2 in]
        n154 = for {
          tunnel: w195 -> [w220] mode=indexing
          tunnel: [w218] -> w194 mode=indexing
          # "Get Plot Names"
          n155 = Format Into String(format string="%.3fGHz", w220) -> (resulting string=w218:string)  [unwired: 2 in, 1 out]
        }
        n156 = Index Array(array=w153, index (row)=1) -> (element=w152:dbl[])  [unwired: 1 in]
        n157 = Index Array(array=w156, index (row)=1) -> (element=w159:dbl[])  [unwired: 1 in]
        n158 = Index Array(array=w158, index (row)=1) -> (element=w161:dbl[])  [unwired: 1 in]
        n159 = Number To Fractional String(number=w152) -> (F-format string=w151:string[])  [unwired: 3 in]
        n160 = Number To Fractional String(number=w159) -> (F-format string=w160:string[])  [unwired: 3 in]
        n161 = Number To Fractional String(number=w161) -> (F-format string=w162:string[])  [unwired: 3 in]
        n162 = local write "Pout@Pin(s)"(w151) -> ()
        n163 = local write "Gain@Pin(s)"(w160) -> ()
        n164 = local write "PAE@Pin(s)"(w162) -> ()
        n165 = local write "Frequencies"(w194) -> ()
      }
      frame "Post UI Update 2" {
        # "---------------Graph5---------------\nPAE vs Pin per Frequency"
        # "---------------Graph2---------------\nLinear Gain vs Frequency"
        # "---------------Graph1---------------\nOPxdB vs Frequency"
        # "---------------Graph4---------------\nGain vs Pin per Frequency"
        # "---------------Graph3---------------\nPout vs Pin per Frequency"
        # "------------------------Table1------------------------\nPout, Gain vs Pin per Freq Graph"
        # "------------------------Table2------------------------\n<Freq><Pin><Pout><Gain><PAE>"
        # "Table1: OPxdB, Gain vs Freq"
        # "Run after Post UI Update. Can be duplicate is need more processing.\nUtilize this case to convert the result to graph or table"
        n166 = local read "Linear Gain vs Freq"() -> (w245:dbl[][])
        n167 = local read "OPxdB vs Freq"() -> (w247:dbl[][])
        n168 = control-ref of="General Graph 1"() -> (w248:refnum<vi>)
        n169 = control-ref of="General Graph 2"() -> (w246:refnum<vi>)
        n170 = Enqueue Element(queue=w257, element="Post UI Update 3", error in (no error)=w259) -> (error out=w258:errorcluster)  [unwired: 1 in, 2 out]
        n171 = call "Graph Assign Plot Names and Data.vi"("Legend Number of Rows"=1, "X Ys Data"=w247, "Graph Ref in"=w248) -> ()  [unwired: 6 in, 3 out]
        n172 = call "Graph Assign Plot Names and Data.vi"("Legend Number of Rows"=1, "X Ys Data"=w245, "Graph Ref in"=w246) -> ()  [unwired: 6 in, 3 out]
        n173 = local read "Table 1 Header"() -> (w224:string[])
        n174 = local read "Linear Gain(s)"() -> (w239:string[])
        n175 = local read "Frequencies"() -> (w241:string[])
        n176 = local read "Pout@Pin(s)"() -> (w223:string[])
        n177 = local read "Gain@Pin(s)"() -> (w222:string[])
        n178 = local read "Pout vs Pin per Freq"() -> (w238:dbl[][])
        n179 = local read "PAE@Pin(s)"() -> (w221:string[])
        n180 = local read "Gain vs Pin per Freq"() -> (w252:dbl[][])
        n181 = local read "OPxdB(s)"() -> (w240:string[])
        n182 = local read "Frequencies"() -> (w232:string[])
        n183 = local read "Frequencies"() -> (w231:string[])
        n184 = control-ref of="MeasTable 1"() -> (w249:refnum<vi>)
        n185 = control-ref of="General Graph 3"() -> (w256:refnum<vi>)
        n186 = control-ref of="General Graph 4"() -> (w253:refnum<vi>)
        n187 = Build Array(w241, w240, w239, w223, w222, w221) -> (w242:string[][])
        n188 = call "Graph Assign Plot Names and Data.vi"("Legend Number of Rows"=5, "X Ys Data"=w238, "Plot Names"=w232, "Graph Ref in"=w256) -> ()  [unwired: 5 in, 3 out]
        n189 = call "Graph Assign Plot Names and Data.vi"("Legend Number of Rows"=5, "X Ys Data"=w252, "Plot Names"=w231, "Graph Ref in"=w253) -> ()  [unwired: 5 in, 3 out]
        n190 = call "Table Set Header Name and Data (String).vi"("Data"=w242, "Header"=w224, "Table Ref"=w249) -> ()  [unwired: 9 in]
        n191 = local read "PAE vs Pin per Freq"() -> (w229:dbl[][])
        n192 = local read "Frequencies"() -> (w230:string[])
        n193 = control-ref of="General Graph 5"() -> (w227:refnum<vi>)
        n194 = call "Graph Assign Plot Names and Data.vi"("Legend Number of Rows"=5, "X Ys Data"=w229, "Plot Names"=w230, "Graph Ref in"=w227) -> ()  [unwired: 5 in, 3 out]
        n195 = local read "Frequencies"() -> (w233:string[])
        n196 = local read "Pin(s)"() -> (w236:string[])
        n197 = Index Array(array=w236) -> (element=w235:string)  [unwired: 1 in]
        n198 = local read "Full Data per Frequency"() -> (w237:string[][])
        n199 = local read "Table 2 Header"() -> (w225:string[])
        n200 = for {
          tunnel: [w261] -> w234 mode=indexing
          tunnel: w235 -> [w261]
          tunnel: w233 -> [_] mode=indexing
        }
        n201 = control-ref of="MeasTable 2"() -> (w251:refnum<vi>)
        n202 = call "Get Data per Frequency at Pin Point Index.vi"("Full Data per Freq"=w237) -> ("Focused Data"=w226:string[][])  [unwired: 10 in]
        n203 = Build Array (concatenate)(w233, w234, w226) -> (w250:string[][])
        n204 = call "Table Set Header Name and Data (String).vi"("Data"=w250, "Header"=w225, "Table Ref"=w251) -> ()  [unwired: 9 in]
      }
      frame "Post UI Update 3" {
        n205 = property on="All Graph Refs" class="Arr (strict)"() -> ("Value"=w266:refnum<vi>[])  [unwired: 2 in, 2 out]
        n206 = call "Graph Cursor Update.vi"("Action"=enum16{"Reset", "Update"}."Update", "error in"=w267, "New X position"=0.0, "Cursor Type"=enum16{"Movable", "Fixed", "All"}."Movable", "Graph Refs in"=w266) -> ("error out"=w262:errorcluster)  [unwired: 5 in, 1 out]
      }
      frame "Exit" {
        # "This case is triggered to close the User Interface from framework"
        n207 = Flush Queue(queue=w272, error in (no error)=w274) -> (queue out=w271:refnum<queue>, error out=w270:errorcluster)  [unwired: 1 out]
        n208 = Release Queue(queue=w271, force destroy? (F)=TRUE, error in (no error)=w270) -> (error out=w269:errorcluster)  [unwired: 2 out]
      }
      frame "Handle Error" {
      }
    }
  }
